vi "FPGA Close.vi"(8 "error in (no error)":errorcluster) -> (0 "error out":errorcluster)   [LabVIEW 2016]
doc: "Closes the FPGA reference."
uses:
  FPGA Global Variables.vi
  <vilib>/FPGAPlugInAG/Dynamic/niLvFpga_Close_Dynamic.vi
  <vilib>/rvi/interface/nirviCloseFPGA/nirviCloseFPGA.xnode
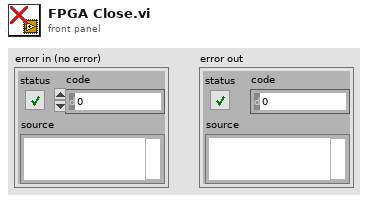
[diagram p1: front panel]
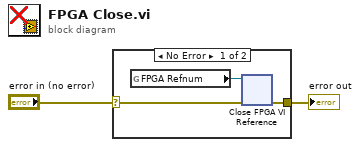
[diagram p0: block diagram]
diagram:
  n1 = case shown="No Error" "error in (no error)" {
    selector: "error in (no error)" -> [w3 w6]
    tunnel: [w4 w6] -> w2
    frame No Error {
      n2 = global read "FPGA Global Variables.vi" "FPGA Refnum"() -> (w5:refnum<k20>)
      n3 = xnode "Close FPGA VI Reference"("FPGA VI Reference In"=w5, "error in"=w3) -> ("error out"=w4:errorcluster)
    }
    frame Error {
    }
  }
  "error out" <- w2
